vi "AB_API Rename Source.vi"(8 "error in (no error)":errorcluster, 9 "New name":string, 10 "source item ID":string, 11 "Build in":refnum<class "AB_Build.lvclass">) -> (0 "error out":errorcluster, 3 "Build out":refnum<class "AB_Build.lvclass">)   [LabVIEW 2020]
uses:
  <vilib>/AppBuilder/AB_Classes/Build/AB_Build.lvclass
  <vilib>/AppBuilder/AB_API/common/AB_API Apply Setting Type.ctl
  <vilib>/AppBuilder/AB_Classes/Source/AB_Source.lvclass
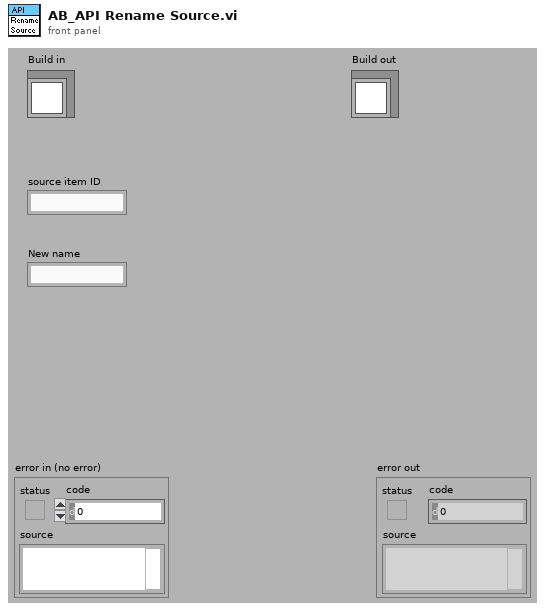
[diagram p1: front panel]
types:
  T1 = typedef "AB_API Apply Setting Type.ctl" = enum16{"Inclusion", "Destination", "Properties", "Password", "Prefix", "SaveSettings"}
  T2 = typedef "AB_Build.ctl" = cluster{"buildSpecName":string, "buildSpecDescription":string, "destinations":refnum<class "AB_Destination.lvclass">[], "exclusionOption":T3, "defaultLanguage":string, "supportedLanguages":string[], "excludedDirectories":path[], "buildContext":refnum<vi>, "buildObject":T4, "preview":bool, "programatic":bool, "progressBarEvents":T5, "userLog_Path":path, "preActionID":string, "preAction_Path":path, "postActionID":string, "postAction_Path":path, "eng_checkForBrokenVIs?":bool, "eng_verboseLinkerErrors?":bool, "localDest_Path":path, "targetDest_Path":path, "removeVIObject":u16, "cache":refnum<class "PreviewCache.lvclass">, "use cache":bool, "previewCache_ID":string, "buildCache_ID":string, "eng_TempLocalDest_Path":path, "eng_collectDependencies?":bool, "versionInfo":cluster{"buildVersion":cluster{"major":u16, "minor":u16, "patch":u16, "build":u16}, "autoIncrement":bool}, "eng_enableVIChecksums":bool}
  T3 = typedef "AB_Exclusion_Option.ctl" = cluster{"typedefs":bool, "polymorphicVIs":bool, "unusedLibraryItems":bool, "modifyLibraryFile":bool, "edit-timeDependencies":bool, "inlineVIs":bool, "dependent PPLs":bool, "dependent DLLs":bool}
  T4 = typedef "ItemRef.ctl" = u64
  T5 = typedef "provcom_ProgressBar_Events.ctl" = cluster{"newJob":refnum<user-event>, "newItem":refnum<user-event>, "errorMsg":T6, "cancel":refnum<user-event>}
  T6 = typedef "mxLvBuildError.ctl" = refnum<user-event>
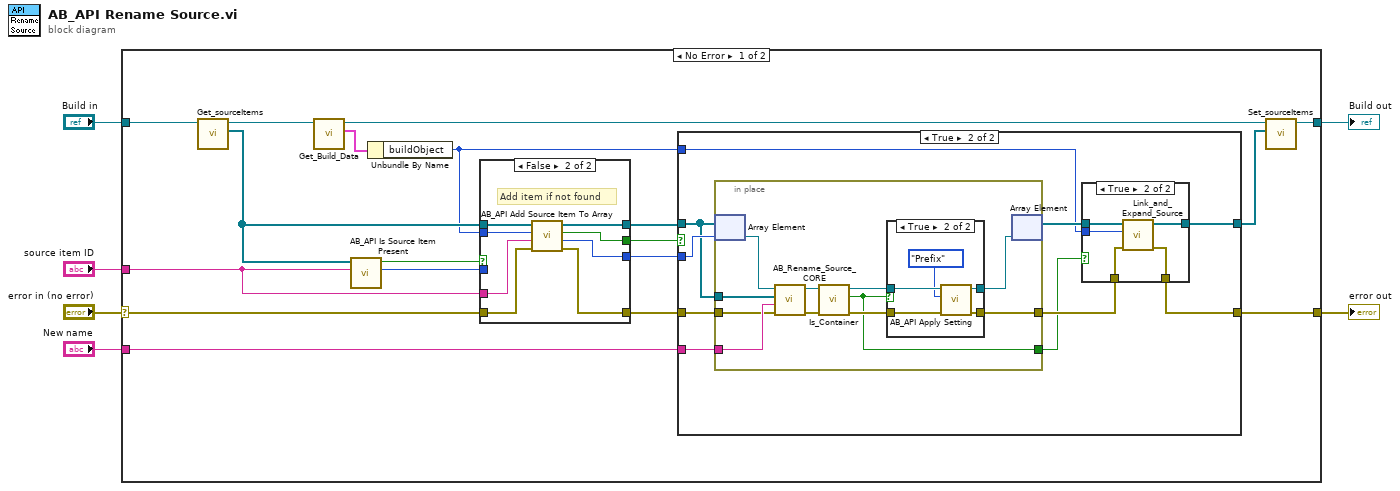
[diagram p0: block diagram]
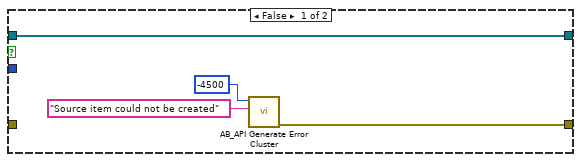
[diagram p3: hidden frame]
diagram:
  n1 = case shown="No Error" "error in (no error)" {
    selector: "error in (no error)" -> [w13 w77]
    tunnel: [w23 w77] -> w5
    tunnel: "New name" -> [w22 _]
    tunnel: "source item ID" -> [w9 _]
    tunnel: "Build in" -> [w21 w76]
    tunnel: [w20 w76] -> w1
    frame No Error {
      n2 = call <vilib>:"Get_sourceItems.vi"("Class in"=w21) -> ("sourceItems"=w17:refnum<class "AB_Source.lvclass">[], "Class out"=w18:refnum<class "AB_Build.lvclass">)  [unwired: 1 in, 8 out]
      n3 = call <vilib>:"Get_Build_Data.vi"("Class in"=w18) -> ("data"=w19:T2, "Class out"=w8:refnum<class "AB_Build.lvclass">)  [unwired: 8 in, 1 out]
      n4 = call <vilib>:"AB_API Is Source Item Present.vi"("item ID"=w9, "source items"=w17) -> ("index"=w14:i32, "source item present?"=w15:bool)  [unwired: 1 in, 7 out]
      n5 = Unbundle By Name(w19) -> ("buildObject"=w7:T4)
      n6 = case shown="False" w15 {
        selector: w15 -> [w28 _]
        tunnel: [w28 w31] -> w10
        tunnel: w14 -> [w27 _]
        tunnel: [w26 w33] -> w12
        tunnel: w13 -> [w26 w34]
        tunnel: [w27 w32] -> w11
        tunnel: w9 -> [_ w29]
        tunnel: [w25 w35] -> w16
        tunnel: w17 -> [w25 w36]
        tunnel: w7 -> [_ w30]
        frame True {
        }
        frame False {
          # "Add item if not found"
          n7 = call <vilib>:"AB_API Add Source Item To Array.vi"("error in (no error)"=w34, "source item ID"=w29, "buildObject"=w30, "source items in"=w36) -> ("error out"=w33:errorcluster, "index"=w32:i32, "added?"=w31:bool, "source items out"=w35:refnum<class "AB_Source.lvclass">[])  [unwired: 4 in]
        }
      }
      n8 = case shown="True" w10 {
        tunnel: w22 -> [_ w50]
        tunnel: [w38 w43] -> w23
        tunnel: w12 -> [_ w47]
        tunnel: w16 -> [w37 w48]
        tunnel: w11 -> [_ w49]
        tunnel: [w37 w45] -> w24
        tunnel: w7 -> [_ w41]
        frame False {
          n9 = call <vilib>:"AB_API Generate Error Cluster.vi"("Additional Message"="Source item could not be created", "Code"=-4500) -> ("error out"=w38:errorcluster)  [unwired: 2 in, 7 out]
        }
        frame True {
          n10 = in-place {
            in-place-border: w50 -> [w66]
            in-place-border: w48 -> [w67]
            in-place-border: w47 -> [w61]
            in-place-border: [w60] -> w44
            in-place-border: [w59] -> w42
            n11 = in-place-array #1(w48, w49) -> (w68:refnum<class "AB_Source.lvclass">)
            n12 = call <vilib>:"AB_Rename_Source_CORE.vi"("error in (no error)"=w61, "New name"=w66, "Source items in"=w67, "Source in"=w68) -> ("error out"=w62:errorcluster, "Source out"=w63:refnum<class "AB_Source.lvclass">)  [unwired: 6 out]
            n13 = call-dynamic "Is_Container.vi"("error in (no error)"=w62, "AB_Source in"=w63) -> ("error out"=w65:errorcluster, "container"=w59:bool, "AB_Source out"=w64:refnum<class "AB_Source.lvclass">)  [unwired: 7 in]
            n14 = case shown="True" w59 {
              tunnel: [w70 w75] -> w58
              tunnel: [w69 w74] -> w60
              tunnel: w64 -> [w70 w73]
              tunnel: w65 -> [w69 w72]
              frame False {
              }
              frame True {
                n15 = call <vilib>:"AB_API Apply Setting.vi"("error in (no error)"=w72, "Settings"=AB_API_Apply_Setting_Type."Prefix", "Source in"=w73) -> ("error out"=w74:errorcluster, "Source out"=w75:refnum<class "AB_Source.lvclass">)  [unwired: 7 in]
              }
            }
            n16 = in-place-array #1(w58) -> (w46:refnum<class "AB_Source.lvclass">[])  [unwired: 1 out]
          }
          n17 = case shown="True" w42 {
            tunnel: w46 -> [w52 w57]
            tunnel: [w52 w56] -> w45
            tunnel: w41 -> [_ w55]
            tunnel: w44 -> [w51 w54]
            tunnel: [w51 w53] -> w43
            frame False {
            }
            frame True {
              n18 = call <vilib>:"Link_and_Expand_Source.vi"("error in (no error)"=w54, "Object"=w55, "AB_Source in"=w57) -> ("error out"=w53:errorcluster, "AB_Source out"=w56:refnum<class "AB_Source.lvclass">[])  [unwired: 7 in]
            }
          }
        }
      }
      n19 = call <vilib>:"Set_sourceItems.vi"("sourceItems"=w24, "Class in"=w8) -> ("Class out"=w20:refnum<class "AB_Build.lvclass">)  [unwired: 1 in, 8 out]
    }
    frame Error {
    }
  }
  "error out" <- w5
  "Build out" <- w1
